vi "总磷总氮测量数据储存.vi"() -> ()   [LabVIEW 2016, in "斯坦道总磷总氮.lvlib"]
uses:
  <vilib>/ptbypt/NI_PtbyPt.lvlib
panel:
  in  "x":bool
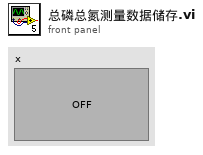
[diagram p1: front panel]
types:
  T1 = cluster{"跨度值":dbl, "零点标准液浓度":dbl, "跨度标准液浓度":dbl, "标准液标准浓度":dbl}
  T2 = cluster{"系统时间":timestamp, "工作状态":u16, "测量模式":enum16{"待机", "连续模式", "周期模式", "定点模式", "受控模式", "手动模式"}, "告警代码":u16, "故障代码":u16, "日志代码":u16, "软件版本":u16, "F0":sgl, "F1":sgl, "F2":sgl, "F3":sgl, "T":sgl, "H":sgl, "id":u16, "flowid":u16, "量程":u16, "总磷控温温度1":sgl, "营养盐控温温度2":sgl, "ADC":sgl, "结果值":sgl, "运行时间":u16, "步骤详情":string, "步骤流程":string}
  T3 = cluster{"运行模式":enum16{"维护模式", "常规模式", "应急模式", "质控模式", "性能测试"}, "质控频次":enum16{"关闭", "每天", "星期一", "星期二", "星期三", "星期四", "星期五", "星期六", "星期日"}, "空白核查时间":u16, "跨度核查时间":u16, "测量间隔":u16}
  T4 = cluster{"因子编码":u32, "单位":u16, "标样参考值":sgl, "水样数据时间":timestamp, "水样实测值":sgl, "水样数据标识":string, "标样数据时间":timestamp, "标样实测值":sgl, "标样数据标识":string, "空白数据时间":timestamp, "空白实测值":sgl, "空白数据标识":string, "零点核查数据时间":timestamp, "零点核查实测值":sgl, "零点核查数据标识":string, "跨度核查数据时间":timestamp, "跨度核查实测值":sgl, "跨度核查数据标识":string, "加标回收数据时间":timestamp, "加标回收实测值":sgl, "加标回收数据标识":string, "平行样数据时间":timestamp, "平行样实测值":sgl, "平行样数据标识":string, "F0":sgl, "F1":sgl, "F2":sgl, "F3":sgl, "F4":sgl, "F5":sgl, "F6":sgl, "F7":sgl, "温度":sgl, "湿度":sgl, "X值":sgl, "fidrange":u16, "X1值":sgl}[]
  T5 = cluster{"总磷跨度值":dbl, "总磷零点标准液浓度":dbl, "总磷跨度标准液浓度":dbl, "总磷标准液标准浓度":dbl, "总氮跨度值":dbl, "总氮零点标准液浓度":dbl, "总氮跨度标准液浓度":dbl, "总氮标准液标准浓度":dbl, "COD跨度值":dbl, "COD零点标准液浓度":dbl, "COD跨度标准液浓度":dbl, "COD标准液标准浓度":dbl, "氨氮跨度值":dbl, "氨氮零点标准液浓度":dbl, "氨氮跨度标准液浓度":dbl, "氨氮标准液标准浓度":dbl, "磷酸盐跨度值":dbl, "磷酸盐零点标准液浓度":dbl, "磷酸盐跨度标准液浓度":dbl, "磷酸盐标准液标准浓度":dbl, "硝氮跨度值":dbl, "硝氮零点标准液浓度":dbl, "硝氮跨度标准液浓度":dbl, "硝氮标准液标准浓度":dbl, "亚硝氮跨度值":dbl, "亚硝氮零点标准液浓度":dbl, "亚硝氮跨度标准液浓度":dbl, "亚硝氮标准液标准浓度":dbl, "硫化物跨度值":dbl, "硫化物零点标准液浓度":dbl, "硫化物跨度标准液浓度":dbl, "硫化物标准液标准浓度":dbl, "硅酸盐跨度值":dbl, "硅酸盐零点标准液浓度":dbl, "硅酸盐跨度标准液浓度":dbl, "硅酸盐标准液标准浓度":dbl, "总磷零点标准液偏差":dbl, "总磷跨度标准液偏差":dbl, "总磷标准液标准偏差":dbl, "总氮零点标准液偏差":dbl, "总氮跨度标准液偏差":dbl, "总氮标准液标准偏差":dbl, "COD零点标准液偏差":dbl, "COD跨度标准液偏差":dbl, "COD标准液标准偏差":dbl, "氨氮零点标准液偏差":dbl, "氨氮跨度标准液偏差":dbl, "氨氮标准液标准偏差":dbl, "磷酸盐零点标准液偏差":dbl, "磷酸盐跨度标准液偏差":dbl, "磷酸盐标准液标准偏差":dbl, "硝氮零点标准液偏差":dbl, "硝氮跨度标准液偏差":dbl, "硝氮标准液标准偏差":dbl, "亚硝氮零点标准液偏差":dbl, "亚硝氮跨度标准液偏差":dbl, "亚硝氮标准液标准偏差":dbl, "硫化物零点标准液偏差":dbl, "硫化物跨度标准液偏差":dbl, "硫化物标准液标准偏差":dbl, "硅酸盐零点标准液偏差":dbl, "硅酸盐跨度标准液偏差":dbl, "硅酸盐标准液标准偏差":dbl, "氟化物跨度值":dbl, "氟化物零点标准液浓度":dbl, "氟化物跨度标准液浓度":dbl, "氟化物标准液标准浓度":dbl, "氟化物零点标准液偏差":dbl, "氟化物跨度标准液偏差":dbl, "氟化物标准液标准偏差":dbl, "CODMn跨度值":dbl, "CODMn零点标准液浓度":dbl, "CODMn跨度标准液浓度":dbl, "CODMn标准液标准浓度":dbl, "CODMn零点标准液偏差":dbl, "CODMn跨度标准液偏差":dbl, "CODMn标准液标准偏差":dbl}
  T6 = enum16{"水样测试", "标样核查", "跨度核查", "零点核查", "加标回收", "空白测试", "平行样"}[]
  T7 = cluster{"因子编码":u32, "单位":u16, "标样参考值":sgl, "水样数据时间":timestamp, "水样实测值":sgl, "水样数据标识":string, "标样数据时间":timestamp, "标样实测值":sgl, "标样数据标识":string, "空白数据时间":timestamp, "空白实测值":sgl, "空白数据标识":string, "零点核查数据时间":timestamp, "零点核查实测值":sgl, "零点核查数据标识":string, "跨度核查数据时间":timestamp, "跨度核查实测值":sgl, "跨度核查数据标识":string, "加标回收数据时间":timestamp, "加标回收实测值":sgl, "加标回收数据标识":string, "平行样数据时间":timestamp, "平行样实测值":sgl, "平行样数据标识":string, "F0":sgl, "F1":sgl, "F2":sgl, "F3":sgl, "F4":sgl, "F5":sgl, "F6":sgl, "F7":sgl, "温度":sgl, "湿度":sgl, "X值":sgl, "fidrange":u16, "X1值":sgl}
  T8 = cluster{"时间标识":timestamp, "测量模式":enum16{"维护数据", "水样测试", "标样核查", "零点核查", "跨度核查", "空白测试", "平行样测试", "加标回收", "空白校准", "标样校准", "初始化（清洗）", "快捷测试"}, "数据标记表":string, "监测值":sgl, "单位":u16, "数据标识":string, "因子编码":u32, "标样参考值":sgl, "F0":sgl, "F1":sgl, "F2":sgl, "F3":sgl, "F4":sgl, "F5":sgl, "F6":sgl, "F7":sgl, "X":sgl, "温度":sgl, "湿度":sgl, "量程标识":string, "SN":string, "跨度值":sgl, "X1":sgl}
  T9 = typedef "斯坦道总磷总氮.lvlib/关键参数.ctl" = cluster{"测量量程":sgl, "测量检出限":sgl, "测量精度":sgl, "测量间隔":sgl, "消解温度":sgl, "消解时长":sgl, "三项式系数":sgl, "二次多项式系数":sgl, "曲线斜率":sgl, "曲线截距":sgl, "线性相关系数":sgl, "空白校准时间":timestamp, "标样校准时间":timestamp, "测量信号值":sgl, "稀释倍数":sgl, "空白标定系数":sgl, "量程系数":sgl}
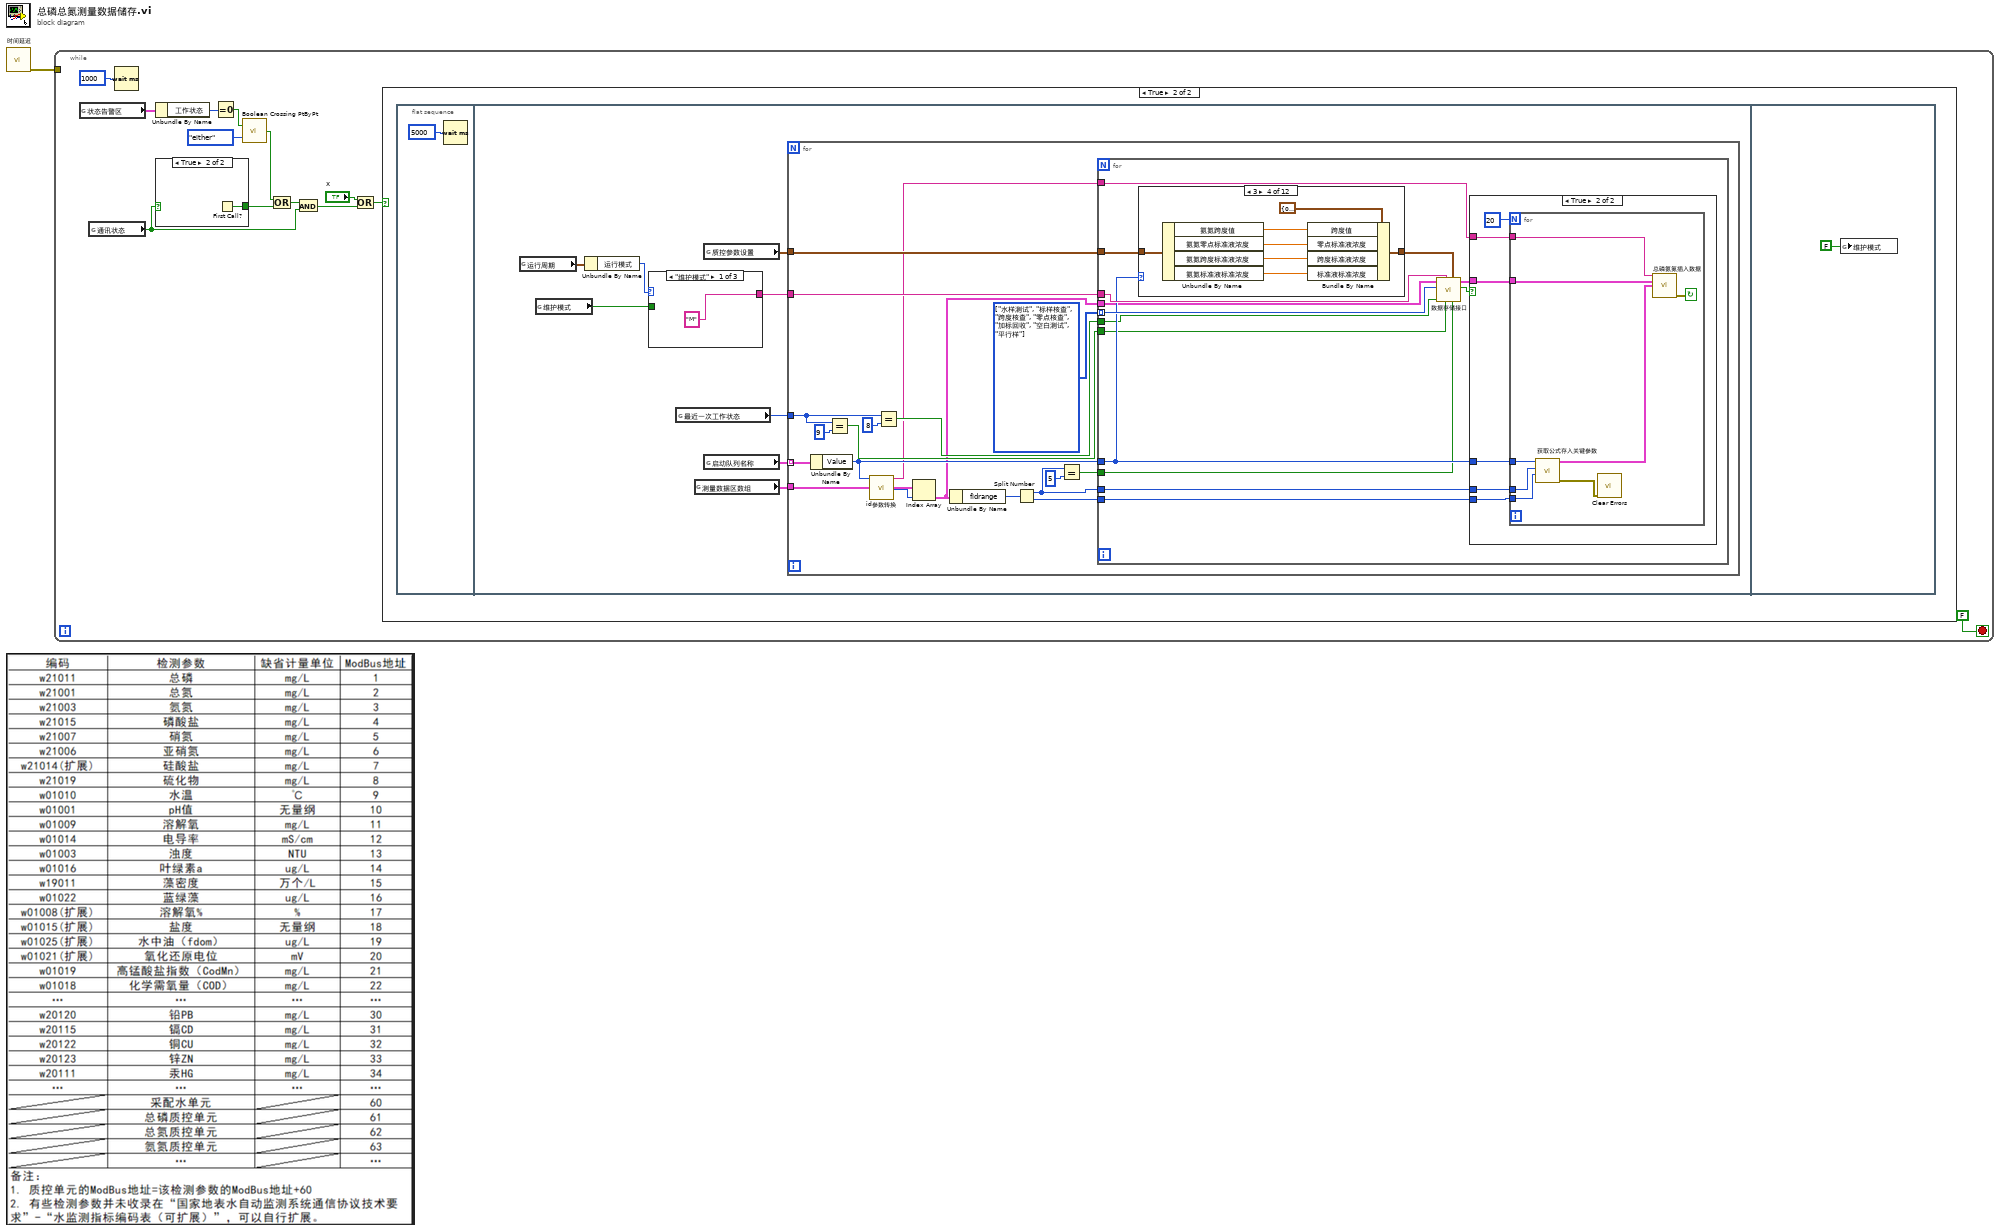
[diagram p0: block diagram]
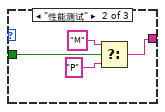
[diagram p4: hidden frame]
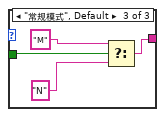
[diagram p5: hidden frame]
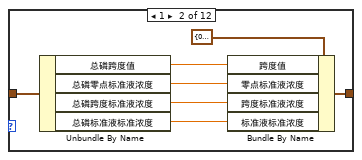
[diagram p8: hidden frame]
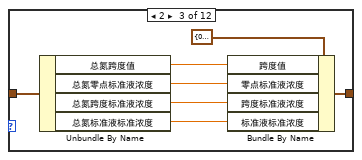
[diagram p9: hidden frame]
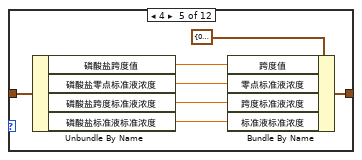
[diagram p10: hidden frame]
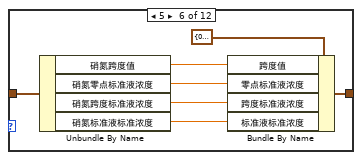
[diagram p11: hidden frame]
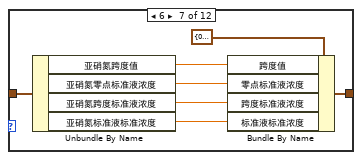
[diagram p12: hidden frame]
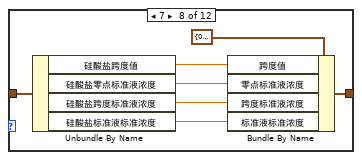
[diagram p13: hidden frame]
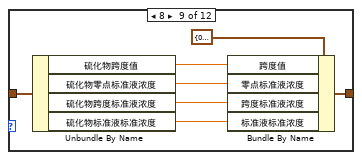
[diagram p14: hidden frame]
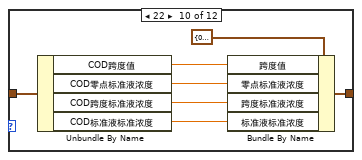
[diagram p15: hidden frame]
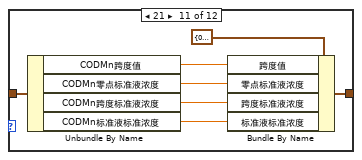
[diagram p16: hidden frame]
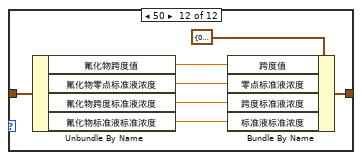
[diagram p17: hidden frame]
diagram:
  n1 = call "时间延迟"() -> ("error out"=w1:errorcluster)  [unwired: 11 in]
  n2 = while {
    tunnel: w1 -> [_]
    stop <- FALSE stop-if-true
    n3 = global read "VAR总磷总氮全局变量.vi" "状态告警区"() -> (w13:T2)
    n4 = global read "VAR总磷总氮全局变量.vi" "通讯状态"() -> (w6:bool)
    n5 = Wait (ms)(milliseconds to wait=u32 1000 ("等待时间（毫秒）")) -> ()  [unwired: 1 out]
    n6 = Unbundle By Name(w13) -> ("工作状态"=w11:u16)
    n7 = case shown="True" w6 {
      tunnel: [_ w15] -> w4
      frame False {
      }
      frame True {
        n8 = First Call?() -> (First Call?: T/F=w15:bool)
      }
    }
    n9 = Equal To 0?(x=w11) -> (x = 0?=w8:bool)
    n10 = call <vilib>:"Boolean Crossing PtByPt.vi"("direction"=enum16{"either", "false-true", "true-false"}."either", "input"=w8) -> ("crossing"=w9:bool)  [unwired: 1 in]
    n11 = Or(x=w9, y=w4) -> (x .or. y?=w5:bool)
    n12 = And(x=w5, y=w6) -> (x .and. y?=w7:bool)
    n13 = Or(x="x", y=w7) -> (x .or. y?=w3:bool)
    n14 = case shown="True" w3 {
      frame False {
      }
      frame True {
        n15 = flat-sequence {
          frame #0 {
            n16 = Wait (ms)(milliseconds to wait=u32 5000 ("等待时间（毫秒）")) -> ()  [unwired: 1 out]
          }
          frame #1 {
            n17 = global read "总磷总氮断电保存全局变量.vi" "运行周期"() -> (w21:T3)
            n18 = global read "VAR总磷总氮全局变量.vi" "维护模式"() -> (w18:bool)
            n19 = Unbundle By Name(w21) -> ("运行模式"=w19:enum16{"维护模式", "常规模式", "应急模式", "质控模式", "性能测试"})
            n20 = case shown="\"维护模式\"" w19 {
              tunnel: ["M" w26 w31] -> w20
              tunnel: w18 -> [_ w27 w33]
              frame "维护模式" {
              }
              frame "性能测试" {
                n21 = Select(t="M", s=w27, f="P") -> (s? t:f=w26:string)
              }
              frame "常规模式", Default {
                n22 = Select(t="M", s=w33, f="N") -> (s? t:f=w31:string)
              }
            }
            n23 = global read "VAR总磷总氮全局变量.vi" "最近一次工作状态"() -> (w23:u16)
            n24 = global read "VAR总磷总氮全局变量.vi" "测量数据区数组"() -> (w17:T4)
            n25 = global read "总磷总氮断电保存全局变量.vi" "质控参数设置"() -> (w22:T5)
            n26 = global read "model config var.vi" "启动队列名称"() -> (w24:cluster{"String":string, "Value":u16}[])
            n27 = for {
              tunnel: w24 -> [w49] mode=indexing
              tunnel: w23 -> [w45]
              tunnel: w22 -> [w51]
              tunnel: w20 -> [w50]
              tunnel: w17 -> [w34]
              w52 = T6 [enum."水样测试", enum."标样核查", enum."跨度核查", enum."零点核查", enum."加标回收", enum."空白测试", enum."平行样"] items=["水样测试", "标样核查", "跨度核查", "零点核查", "加标回收", "空白测试", "平行样"]
              n28 = Unbundle By Name(w49) -> ("Value"=w43:u16)
              n29 = Equal?(x=w45, y=u16 9) -> (x = y?=w44:bool)
              n30 = call "id参数转换.vi"("id"=w43) -> ("table输出"=w42:string, "数组资源索引"=w35:i32)  [unwired: 9 in]
              n31 = Equal?(x=w45, y=u16 8) -> (x = y?=w47:bool)
              n32 = Index Array(array=w34, index=w35) -> (element=w39:T7)
              n33 = Unbundle By Name(w39) -> ("fidrange"=w41:u16)
              n34 = Split Number(x=w41) -> (hi(x)=w36:u8, lo(x)=w37:u8)
              n35 = Equal?(x=w36, y=u16 5) -> (x = y?=w38:bool)
              n36 = for {
                tunnel: w52 -> [w64] mode=indexing
                tunnel: w51 -> [w63]
                tunnel: w50 -> [w62]
                tunnel: w43 -> [w61]
                tunnel: w47 -> [w60]
                tunnel: w44 -> [w59]
                tunnel: w39 -> [w54]
                tunnel: w42 -> [w58]
                tunnel: w38 -> [w57]
                tunnel: w37 -> [w56]
                tunnel: w36 -> [w55]
                n37 = case shown="3" w61 {
                  tunnel: w63 -> [_ w87 w94 w101 w108 w115 w122 w129 w136 w143 w150 w157]
                  tunnel: [_ w85 w92 w99 w106 w113 w120 w127 w134 w141 w148 w155] -> w65
                  frame 0, Default {
                  }
                  frame 1 {
                    n38 = Unbundle By Name(w87) -> ("总磷跨度值"=w84:dbl, "总磷零点标准液浓度"=w83:dbl, "总磷跨度标准液浓度"=w82:dbl, "总磷标准液标准浓度"=w81:dbl)
                    n39 = Bundle By Name(cluster=T1 {"跨度值"=0.0, "零点标准液浓度"=0.0, "跨度标准液浓度"=0.0, "标准液标准浓度"=0.0} ("质控参数设置"), "跨度值"=w84, "零点标准液浓度"=w83, "跨度标准液浓度"=w82, "标准液标准浓度"=w81) -> (w85:T1)
                  }
                  frame 2 {
                    n40 = Unbundle By Name(w94) -> ("总氮跨度值"=w91:dbl, "总氮零点标准液浓度"=w90:dbl, "总氮跨度标准液浓度"=w89:dbl, "总氮标准液标准浓度"=w88:dbl)
                    n41 = Bundle By Name(cluster=T1 {"跨度值"=0.0, "零点标准液浓度"=0.0, "跨度标准液浓度"=0.0, "标准液标准浓度"=0.0} ("质控参数设置"), "跨度值"=w91, "零点标准液浓度"=w90, "跨度标准液浓度"=w89, "标准液标准浓度"=w88) -> (w92:T1)
                  }
                  frame 3 {
                    n42 = Unbundle By Name(w101) -> ("氨氮跨度值"=w98:dbl, "氨氮零点标准液浓度"=w97:dbl, "氨氮跨度标准液浓度"=w96:dbl, "氨氮标准液标准浓度"=w95:dbl)
                    n43 = Bundle By Name(cluster=T1 {"跨度值"=0.0, "零点标准液浓度"=0.0, "跨度标准液浓度"=0.0, "标准液标准浓度"=0.0} ("质控参数设置"), "跨度值"=w98, "零点标准液浓度"=w97, "跨度标准液浓度"=w96, "标准液标准浓度"=w95) -> (w99:T1)
                  }
                  frame 4 {
                    n44 = Unbundle By Name(w108) -> ("磷酸盐跨度值"=w105:dbl, "磷酸盐零点标准液浓度"=w104:dbl, "磷酸盐跨度标准液浓度"=w103:dbl, "磷酸盐标准液标准浓度"=w102:dbl)
                    n45 = Bundle By Name(cluster=T1 {"跨度值"=0.0, "零点标准液浓度"=0.0, "跨度标准液浓度"=0.0, "标准液标准浓度"=0.0} ("质控参数设置"), "跨度值"=w105, "零点标准液浓度"=w104, "跨度标准液浓度"=w103, "标准液标准浓度"=w102) -> (w106:T1)
                  }
                  frame 5 {
                    n46 = Unbundle By Name(w115) -> ("硝氮跨度值"=w112:dbl, "硝氮零点标准液浓度"=w111:dbl, "硝氮跨度标准液浓度"=w110:dbl, "硝氮标准液标准浓度"=w109:dbl)
                    n47 = Bundle By Name(cluster=T1 {"跨度值"=0.0, "零点标准液浓度"=0.0, "跨度标准液浓度"=0.0, "标准液标准浓度"=0.0} ("质控参数设置"), "跨度值"=w112, "零点标准液浓度"=w111, "跨度标准液浓度"=w110, "标准液标准浓度"=w109) -> (w113:T1)
                  }
                  frame 6 {
                    n48 = Unbundle By Name(w122) -> ("亚硝氮跨度值"=w119:dbl, "亚硝氮零点标准液浓度"=w118:dbl, "亚硝氮跨度标准液浓度"=w117:dbl, "亚硝氮标准液标准浓度"=w116:dbl)
                    n49 = Bundle By Name(cluster=T1 {"跨度值"=0.0, "零点标准液浓度"=0.0, "跨度标准液浓度"=0.0, "标准液标准浓度"=0.0} ("质控参数设置"), "跨度值"=w119, "零点标准液浓度"=w118, "跨度标准液浓度"=w117, "标准液标准浓度"=w116) -> (w120:T1)
                  }
                  frame 7 {
                    n50 = Unbundle By Name(w129) -> ("硅酸盐跨度值"=w126:dbl, "硅酸盐零点标准液浓度"=w125:dbl, "硅酸盐跨度标准液浓度"=w124:dbl, "硅酸盐标准液标准浓度"=w123:dbl)
                    n51 = Bundle By Name(cluster=T1 {"跨度值"=0.0, "零点标准液浓度"=0.0, "跨度标准液浓度"=0.0, "标准液标准浓度"=0.0} ("质控参数设置"), "跨度值"=w126, "零点标准液浓度"=w125, "跨度标准液浓度"=w124, "标准液标准浓度"=w123) -> (w127:T1)
                  }
                  frame 8 {
                    n52 = Unbundle By Name(w136) -> ("硫化物跨度值"=w133:dbl, "硫化物零点标准液浓度"=w132:dbl, "硫化物跨度标准液浓度"=w131:dbl, "硫化物标准液标准浓度"=w130:dbl)
                    n53 = Bundle By Name(cluster=T1 {"跨度值"=0.0, "零点标准液浓度"=0.0, "跨度标准液浓度"=0.0, "标准液标准浓度"=0.0} ("质控参数设置"), "跨度值"=w133, "零点标准液浓度"=w132, "跨度标准液浓度"=w131, "标准液标准浓度"=w130) -> (w134:T1)
                  }
                  frame 22 {
                    n54 = Unbundle By Name(w143) -> ("COD跨度值"=w140:dbl, "COD零点标准液浓度"=w139:dbl, "COD跨度标准液浓度"=w138:dbl, "COD标准液标准浓度"=w137:dbl)
                    n55 = Bundle By Name(cluster=T1 {"跨度值"=0.0, "零点标准液浓度"=0.0, "跨度标准液浓度"=0.0, "标准液标准浓度"=0.0} ("质控参数设置"), "跨度值"=w140, "零点标准液浓度"=w139, "跨度标准液浓度"=w138, "标准液标准浓度"=w137) -> (w141:T1)
                  }
                  frame 21 {
                    n56 = Unbundle By Name(w150) -> ("CODMn跨度值"=w147:dbl, "CODMn零点标准液浓度"=w146:dbl, "CODMn跨度标准液浓度"=w145:dbl, "CODMn标准液标准浓度"=w144:dbl)
                    n57 = Bundle By Name(cluster=T1 {"跨度值"=0.0, "零点标准液浓度"=0.0, "跨度标准液浓度"=0.0, "标准液标准浓度"=0.0} ("质控参数设置"), "跨度值"=w147, "零点标准液浓度"=w146, "跨度标准液浓度"=w145, "标准液标准浓度"=w144) -> (w148:T1)
                  }
                  frame 50 {
                    n58 = Unbundle By Name(w157) -> ("氟化物跨度值"=w154:dbl, "氟化物零点标准液浓度"=w153:dbl, "氟化物跨度标准液浓度"=w152:dbl, "氟化物标准液标准浓度"=w151:dbl)
                    n59 = Bundle By Name(cluster=T1 {"跨度值"=0.0, "零点标准液浓度"=0.0, "跨度标准液浓度"=0.0, "标准液标准浓度"=0.0} ("质控参数设置"), "跨度值"=w154, "零点标准液浓度"=w153, "跨度标准液浓度"=w152, "标准液标准浓度"=w151) -> (w155:T1)
                  }
                }
                n60 = call "数据存储接口.vi"("快捷测试？"=w57, "质控参数设置"=w65, "标样校准？"=w59, "数据标记表"=w62, "空白校准？"=w60, "数据存储模式"=w64, "测量数据区"=w54) -> ("x != y?"=w53:bool, "data输出"=w66:T8)  [unwired: 3 in]
                n61 = case shown="True" w53 {
                  tunnel: w66 -> [_ w72]
                  tunnel: w61 -> [_ w71]
                  tunnel: w58 -> [_ w70]
                  tunnel: w56 -> [_ w69]
                  tunnel: w55 -> [_ w68]
                  frame False {
                  }
                  frame True {
                    n62 = for {
                      N: 20 -> [_]
                      tunnel: w72 -> [w80]
                      tunnel: w71 -> [w78]
                      tunnel: w70 -> [w77]
                      tunnel: w69 -> [w76]
                      tunnel: w68 -> [w75]
                      stop <- w74 continue-if-true
                      n63 = call "获取公式存入关键参数.vi"("量程"=w76, "flowid"=w75, "id"=w78) -> ("error out"=w73:errorcluster, "关键参数"=w79:T9)  [unwired: 7 in]
                      n64 = call <vilib>:"Clear Errors.vi"("error in (no error)"=w73) -> ()  [unwired: 5 in, 2 out]
                      n65 = call "总磷氨氮插入数据.vi"("table"=w77, "data"=w80, "关键参数"=w79) -> ("error out"=w74:errorcluster)  [unwired: 12 in]
                    }
                  }
                }
              }
            }
          }
          frame #2 {
            n66 = global write "VAR总磷总氮全局变量.vi" "维护模式"(FALSE ("维护模式")) -> ()
          }
        }
      }
    }
  }
